vi "LOC subReadWriteVIStringINIKeys(String Array).vi"(4 "Mode":enum16{"Read", "Write"}(ring), 5 "Section":string, 6 "error in (no error)":errorcluster, 8 "ConfigFileRefnum":T1, 9 "ControlRefnum":refnum<vi>) -> (0 "error out":errorcluster)   [LabVIEW 2020, in "Localization_Tools.lvlib"]
uses:
  Localization_Tools.lvlib
  <vilib>/Utility/config.llb/Config Data RefNum.ctl
  <vilib>/Utility/config.llb/NI_LVConfig.lvlib
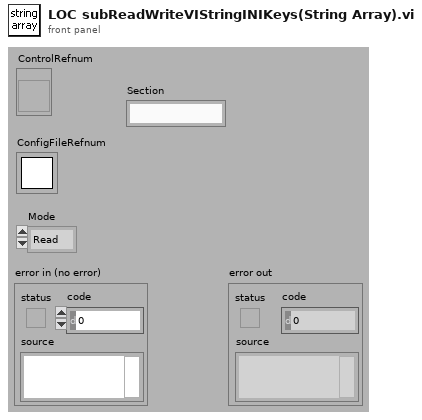
[diagram p1: front panel]
types:
  T1 = typedef "NI_LVConfig.lvlib/Config Data RefNum.ctl" = refnum<k1>
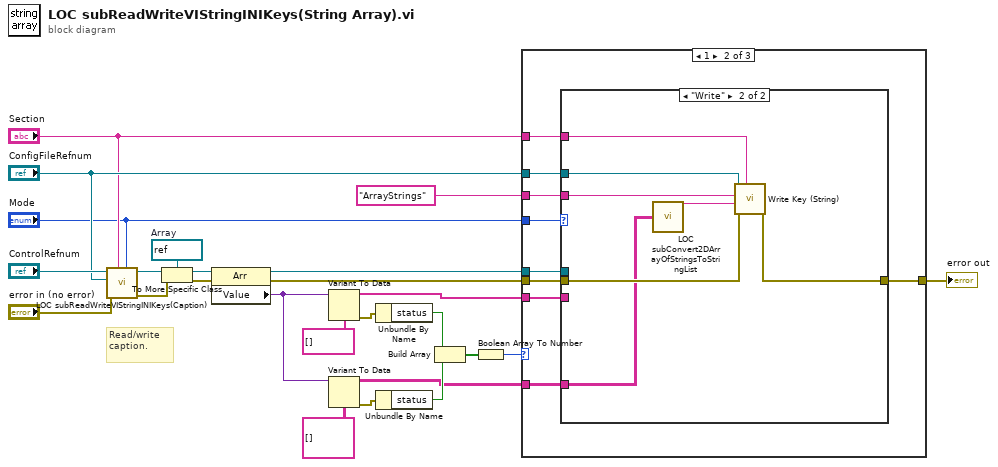
[diagram p0: block diagram]
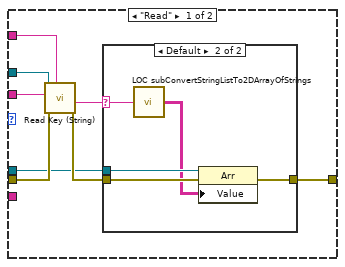
[diagram p3: hidden frame]
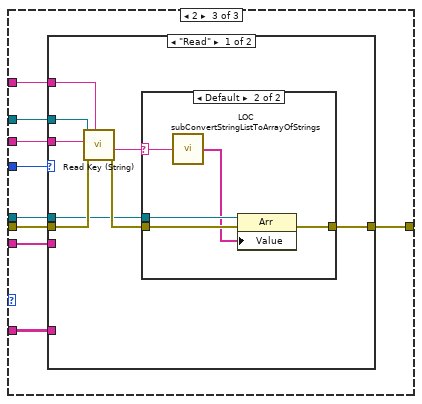
[diagram p5: hidden frame]
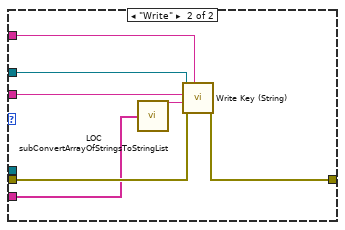
[diagram p7: hidden frame]
diagram:
  w18 = refnum<vi> refnum  # Array
  # "Read/write\ncaption."
  n1 = call "LOC subReadWriteVIStringINIKeys(Caption).vi"("Mode"="Mode", "Section"="Section", "error in (no error)"="error in (no error)", "ConfigFileRefnum"="ConfigFileRefnum", "ControlRefnum"="ControlRefnum") -> ("error out"=w16:errorcluster, "dup ControlRefnum"=w17:refnum<vi>)  [unwired: 3 in]
  n2 = To More Specific Class(target class=w18, reference=w17, error in=w16) -> (specific class reference=w15:refnum<vi>, error out=w14:errorcluster)
  n3 = property class="Arr"(reference=w15, error in=w14) -> (reference out=w12:refnum<vi>, error out=w13:errorcluster, "Value"=w11:variant)
  n4 = Variant To Data(type=string[] [], Variant=w11) -> (data=w2:string[], error out=w8:errorcluster)  [unwired: 1 in]
  n5 = Variant To Data(type=string[][] [], Variant=w11) -> (data=w1:string[][], error out=w7:errorcluster)  [unwired: 1 in]
  n6 = Unbundle By Name(w8) -> ("status"=w6:bool)
  n7 = Unbundle By Name(w7) -> ("status"=w5:bool)
  n8 = Build Array(w6, w5) -> (w4:bool[])
  n9 = Boolean Array To Number(Boolean array=w4) -> (number=w3:u32)
  n10 = case shown="1" w3 {
    tunnel: "ArrayStrings" ("key") -> [_ w35 w65]
    tunnel: "ConfigFileRefnum" -> [_ w34 w64]
    tunnel: "Section" -> [_ w33 w63]
    tunnel: "Mode" -> [_ w32 w62]
    tunnel: [w26 w31 w61] -> w19
    tunnel: w13 -> [w26 w30 w60]
    tunnel: w12 -> [_ w29 w59]
    tunnel: w2 -> [_ w28 w58]
    tunnel: w1 -> [_ w27 w57]
    frame 0, 3, Default {
    }
    frame 1 {
      n11 = case shown="\"Write\"" w32 {
        tunnel: w29 -> [w37 _]
        tunnel: w30 -> [w38 w52]
        tunnel: w34 -> [w43 w56]
        tunnel: w33 -> [w42 w54]
        tunnel: w35 -> [w41 w55]
        tunnel: [w39 w53] -> w31
        tunnel: w28 -> [_ _]
        tunnel: w27 -> [_ w50]
        frame "Read" {
          n12 = call <vilib>:"Read Key (String).vi"("section"=w42, "error in (no error)"=w38, "key"=w41, "refnum"=w43) -> ("error out"=w40:errorcluster, "value"=w36:string)  [unwired: 4 in, 2 out]
          n13 = case shown="Default" w36 {
            selector: w36 -> [_ w45]
            tunnel: w40 -> [w44 w49]
            tunnel: [w44 w48] -> w39
            tunnel: w37 -> [_ w47]
            frame "" {
            }
            frame Default {
              n14 = call "LOC subConvertStringListTo2DArrayOfStrings.vi"("InputString"=w45) -> ("OutputArray"=w46:string[][])
              n15 = property class="Arr"(reference=w47, error in=w49, "Value"=w46) -> (error out=w48:errorcluster)  [unwired: 1 out]
            }
          }
        }
        frame "Write" {
          n16 = call "LOC subConvert2DArrayOfStringsToStringList.vi"("InputArray"=w50) -> ("OutputString"=w51:string)
          n17 = call <vilib>:"Write Key (String).vi"("section"=w54, "error in (no error)"=w52, "value"=w51, "key"=w55, "refnum"=w56) -> ("error out"=w53:errorcluster)  [unwired: 4 in, 2 out]
        }
      }
    }
    frame 2 {
      n18 = case shown="\"Read\"" w62 {
        tunnel: w59 -> [w67 _]
        tunnel: w60 -> [w68 w82]
        tunnel: w64 -> [w73 w86]
        tunnel: w63 -> [w72 w84]
        tunnel: w65 -> [w71 w85]
        tunnel: [w69 w83] -> w61
        tunnel: w58 -> [_ w80]
        tunnel: w57 -> [_ _]
        frame "Read" {
          n19 = call <vilib>:"Read Key (String).vi"("section"=w72, "error in (no error)"=w68, "key"=w71, "refnum"=w73) -> ("error out"=w70:errorcluster, "value"=w66:string)  [unwired: 4 in, 2 out]
          n20 = case shown="Default" w66 {
            selector: w66 -> [_ w75]
            tunnel: w70 -> [w74 w79]
            tunnel: [w74 w78] -> w69
            tunnel: w67 -> [_ w77]
            frame "" {
            }
            frame Default {
              n21 = call "LOC subConvertStringListToArrayOfStrings.vi"("InputString"=w75) -> ("OutputArray"=w76:string[])
              n22 = property class="Arr"(reference=w77, error in=w79, "Value"=w76) -> (error out=w78:errorcluster)  [unwired: 1 out]
            }
          }
        }
        frame "Write" {
          n23 = call "LOC subConvertArrayOfStringsToStringList.vi"("InputArray"=w80) -> ("OutputString"=w81:string)
          n24 = call <vilib>:"Write Key (String).vi"("section"=w84, "error in (no error)"=w82, "value"=w81, "key"=w85, "refnum"=w86) -> ("error out"=w83:errorcluster)  [unwired: 4 in, 2 out]
        }
      }
    }
  }
  "error out" <- w19
